vi "ComponentSimulatorA.vi"(8 "error in":errorcluster, 10 "ServerConfiguration":T1={"cmdServerPort"=8888, "telServerPort"=8889, "timeoutServerInMs"=100, "serverBytesToRead"=32768, "maxSizeQueueTcpClientFromDds"=1000, "EnqueueOptions"=enum."lossy enqueue", "timeoutQueueTcpClientFromDds (ms)"=50, "maxSizeQueueTcpClient"=1000, "timeoutInMs"=100}, 11 "tcpServer in":refnum<class "TcpServer.lvclass">) -> (0 "error out":errorcluster)   [LabVIEW 2018]
doc: "Simulate a software component that will use the TCP Server."
uses:
  src/TcpServerTel/typedef/queueOptionsTypeDef.ctl
  src/TcpServerTel/typedef/enqueueOptionsTypeDef.ctl
  src/TcpServer/configServerTypeDef.ctl
  src/TcpServer/TcpServer.lvclass
  src/TcpServerTel/typedef/telTypeDef.ctl
  src/TcpServer/TcpServer.lvclass/TcpServer.ctl
  src/TcpServerTel/TcpServerTel.lvclass/TcpServerTel.ctl
  src/TcpServer/runServer.vi
  src/TcpServerTel/TcpServerTel.lvclass
panel:
  out "Generic Message":string
  out "Clients Connected":bool
  in  "Telemetry Options":T3={"EnqueueOptions"=enum."lossy enqueue", "Timeout (ms)"=50}
  in  "Telemetry Timeout (ms)":i32=50
  out "Remaining Elements":i32
  out "One instance telemetry":string
  in  "getOneInstance":bool
  out "Telemetry Flushed":string[](array[string])
  in  "getQueueSize":bool
  out "Queue Size":i32
  in  "flushQueueFromDds":bool
  out "Event Received":string
  out "Command Received":string
  in  "Tab Control":T4(tab)
  out "ServerConfiguration":T1={"cmdServerPort"=8888, "telServerPort"=8889, "timeoutServerInMs"=100, "serverBytesToRead"=32768, "maxSizeQueueTcpClientFromDds"=1000, "EnqueueOptions"=enum."lossy enqueue", "timeoutQueueTcpClientFromDds (ms)"=50, "maxSizeQueueTcpClient"=1000, "timeoutInMs"=100}
  in  "fail":bool
  in  "success":bool
  in  "send_event":bool
  in  "Event Id":string="move"
  in  "Event Details":string="\"InPosition\" : true\n\n\"Tolerance\" : 0.2"
  in  "flushQueueToDds":bool
  in  "isQueueFull":bool
  in  "publish_telemetry":bool
  in  "send_telemetry":bool
  in  "Frecuency (cycles/s)":dbl=10.0
  in  "Duration (s)":dbl=2.0
  out "queueToDds":bool
  in  "Telemetry":T5={"Telemetry Id"="elevation", "telDetails"="\"compName\":\"MTMount\""}
  in  "stop_server":bool
  in  "Stop Simulator":bool caption="stop"
  # "Component Simulator A"
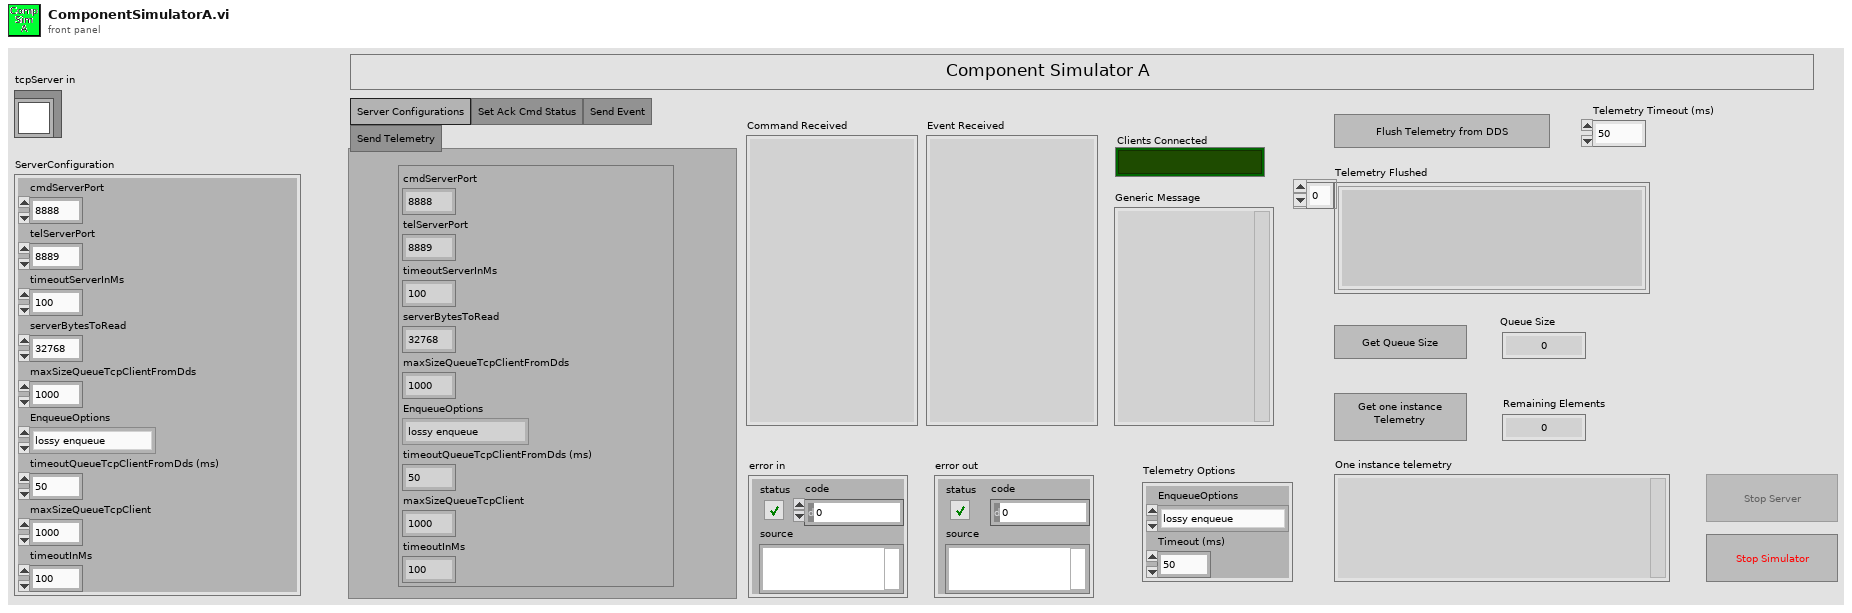
[diagram p1: front panel]
types:
  T1 = typedef "TcpServer.lvclass/configServerTypeDef.ctl" = cluster{"cmdServerPort":u16, "telServerPort":u16, "timeoutServerInMs":i32, "serverBytesToRead":i32, "maxSizeQueueTcpClientFromDds":i32, "EnqueueOptions":T2, "timeoutQueueTcpClientFromDds (ms)":i32, "maxSizeQueueTcpClient":i32, "timeoutInMs":i32}
  T2 = typedef "TcpServerTel.lvclass/enqueueOptionsTypeDef.ctl" = enum16{"lossy enqueue", "normal enqueue"}
  T3 = typedef "TcpServerTel.lvclass/queueOptionsTypeDef.ctl" = cluster{"EnqueueOptions":T2, "Timeout (ms)":i32}
  T4 = enum32{"Server Configurations", "Set Ack Cmd Status", "Send Event", "Send Telemetry"}
  T5 = cluster{"Telemetry Id":string, "telDetails":string}
  T6 = typedef "TcpServerTel.lvclass/telTypeDef.ctl" = cluster{"name":string, "telDetails":string}
  T7 = enum16{"queueTcpClientFromDds", "queueTcpClient"}
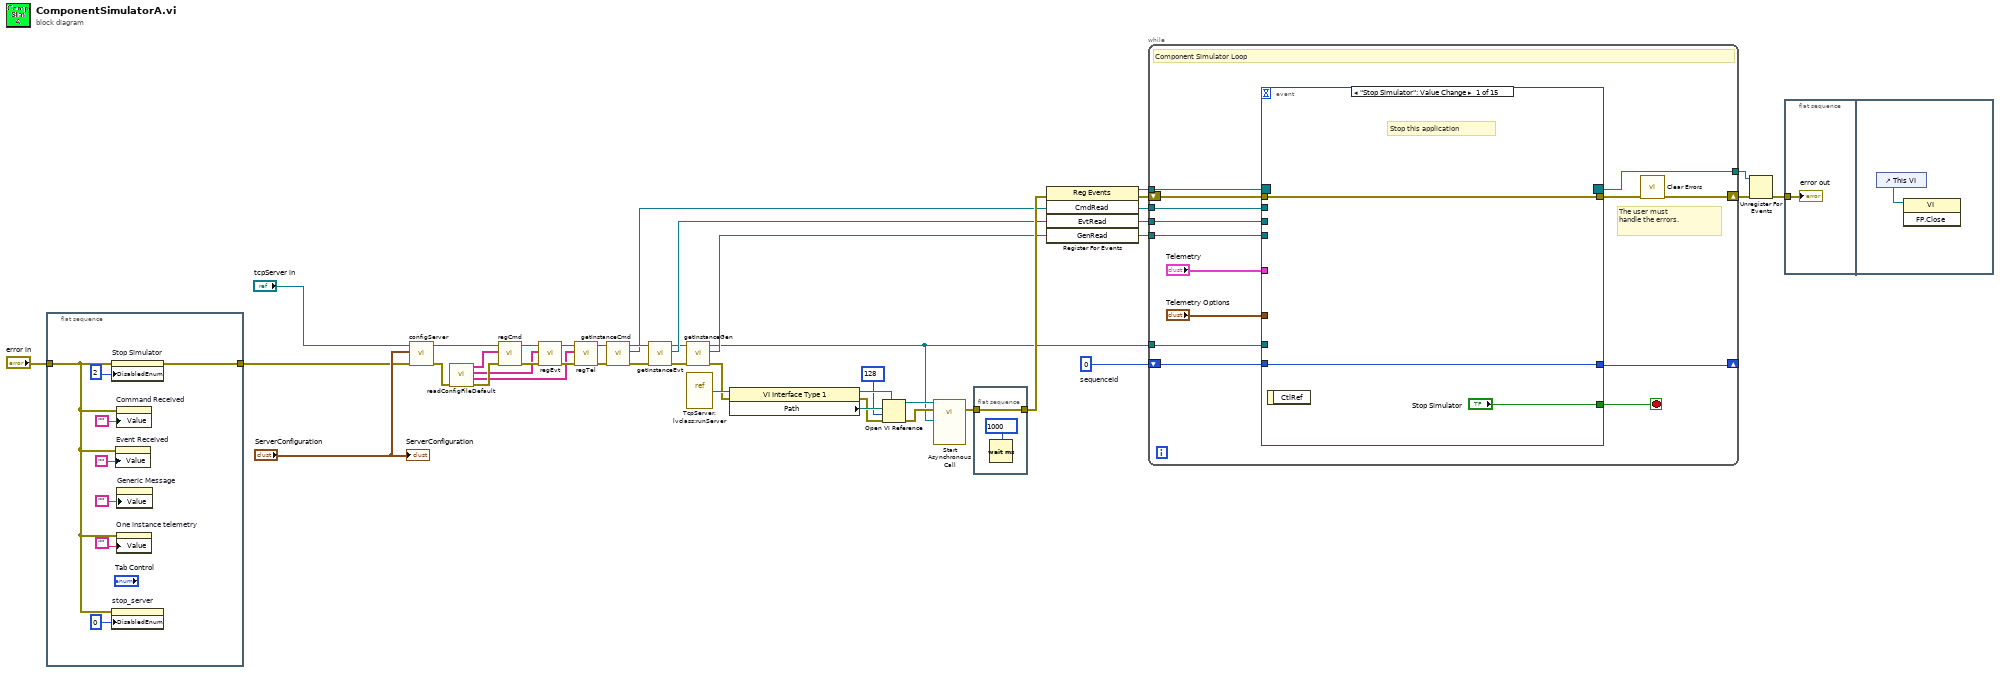
[diagram p0: block diagram]
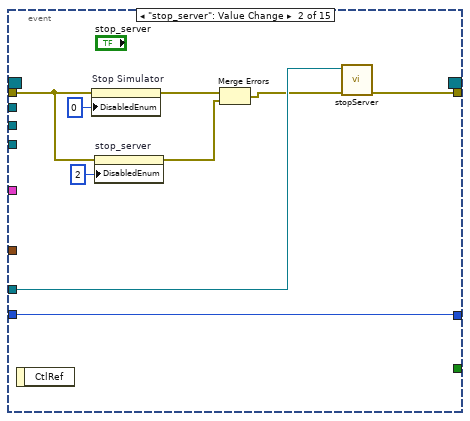
[diagram p2: hidden frame]
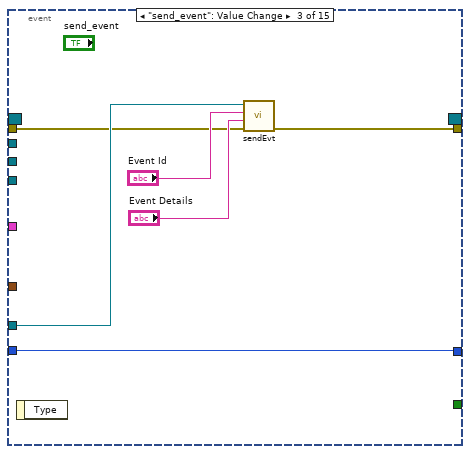
[diagram p3: hidden frame]
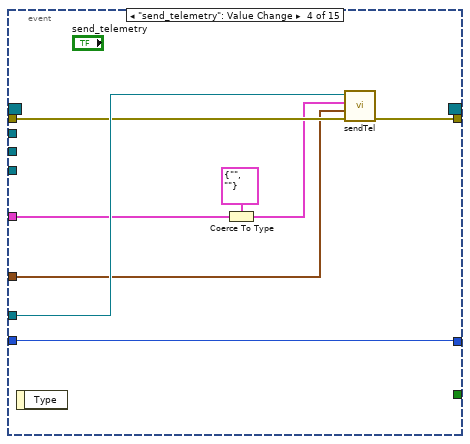
[diagram p4: hidden frame]
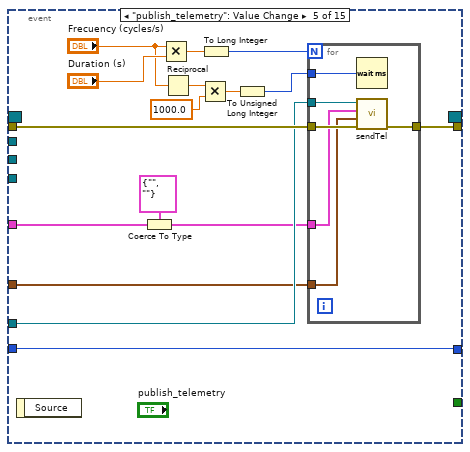
[diagram p5: hidden frame]
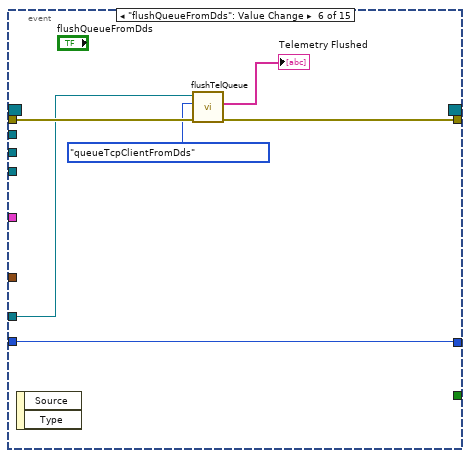
[diagram p6: hidden frame]
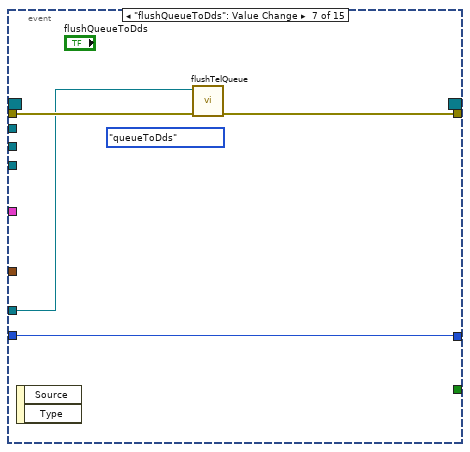
[diagram p7: hidden frame]
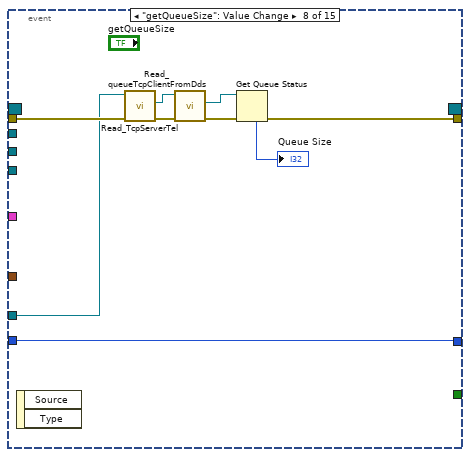
[diagram p8: hidden frame]
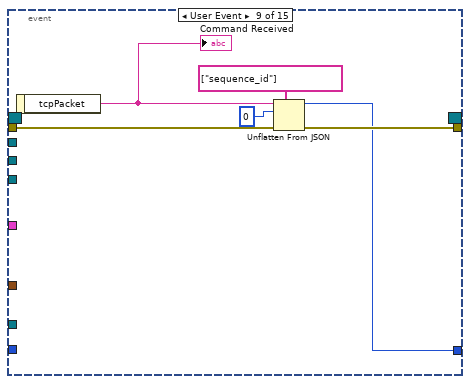
[diagram p9: hidden frame]
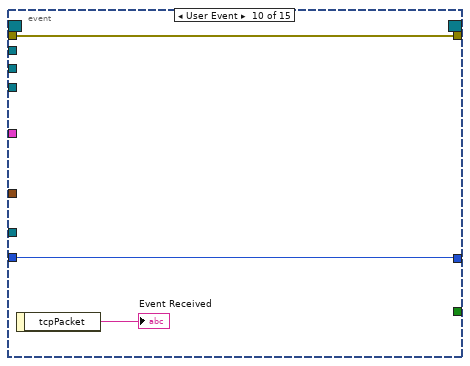
[diagram p10: hidden frame]
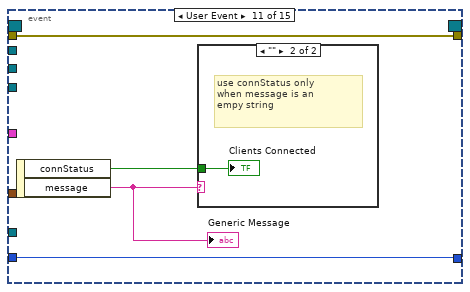
[diagram p11: hidden frame]
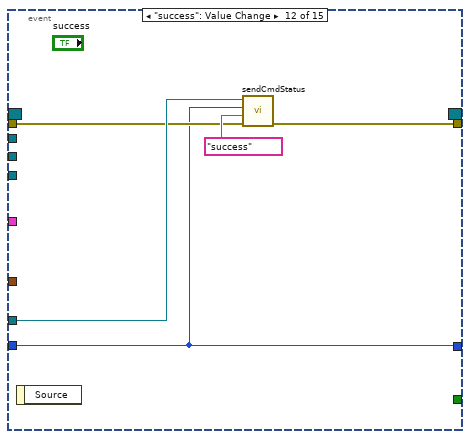
[diagram p13: hidden frame]
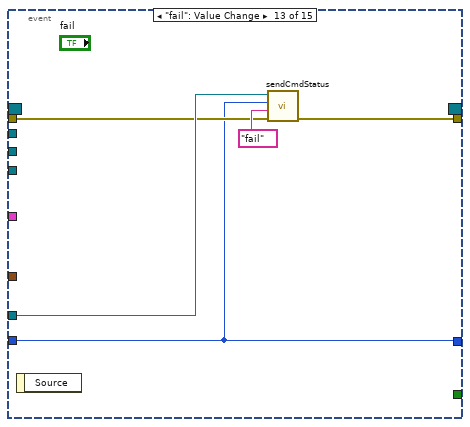
[diagram p14: hidden frame]
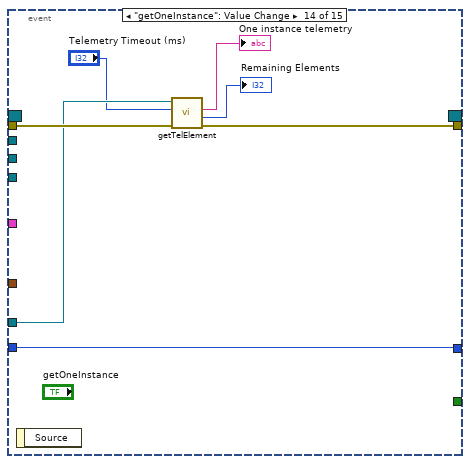
[diagram p15: hidden frame]
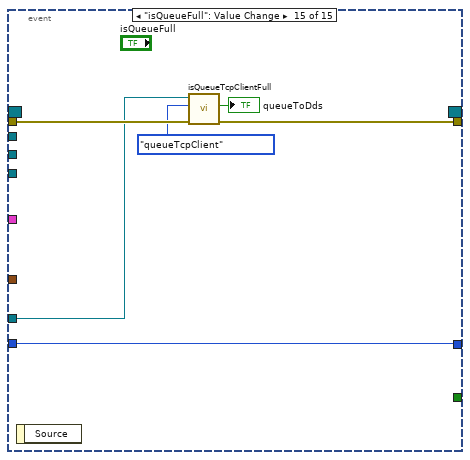
[diagram p16: hidden frame]
diagram:
  w5 = 0  # sequenceId
  n1 = flat-sequence {
    tunnel: "error in" -> [w43]
    tunnel: [w47] -> w2
    frame #0 {
      n2 = property on="Stop Simulator" class="Bool"(error in=w43, "DisabledEnum"=2) -> (error out=w47:errorcluster)  [unwired: 1 in, 1 out]
      n3 = property on="stop_server" class="Bool"(error in=w43, "DisabledEnum"=0) -> ()  [unwired: 1 in, 2 out]
      n4 = property on="Event Received" class="Str"(error in=w43, "Value"="") -> ()  [unwired: 1 in, 2 out]
      n5 = property on="Command Received" class="Str"(error in=w43, "Value"="") -> ()  [unwired: 1 in, 2 out]
      n6 = property on="One instance telemetry" class="Str"(error in=w43, "Value"="") -> ()  [unwired: 1 in, 2 out]
      n7 = property on="Generic Message" class="Str"("Value"="") -> ()  [unwired: 2 in, 2 out]
    }
  }
  n8 = call "configServer.vi"("error in (no error)"=w2, "ServerConfiguration"="ServerConfiguration", "tcpServer in"="tcpServer in") -> ("error out"=w14:errorcluster, "tcpServer out"=w37:refnum<class "TcpServer.lvclass">)  [unwired: 7 in]
  n9 = call "readConfigFileDefault.vi"("error in (no error)"=w14) -> ("error out"=w13:errorcluster, "regTel"=w7:string[][], "regEvt"=w11:string[][], "regCmd"=w12:string[])  [unwired: 7 in]
  n10 = call "regCmd.vi"("error in (no error)"=w13, "cmdReg"=w12, "tcpServer in"=w37) -> ("error out"=w38:errorcluster, "tcpServer out"=w18:refnum<class "TcpServer.lvclass">)  [unwired: 7 in]
  n11 = call "regEvt.vi"("error in (no error)"=w38, "evtReg"=w11, "tcpServer in"=w18) -> ("error out"=w19:errorcluster, "tcpServer out"=w9:refnum<class "TcpServer.lvclass">)  [unwired: 7 in]
  n12 = call "regTel.vi"("error in (no error)"=w19, "telReg"=w7, "tcpServer in"=w9) -> ("error out"=w10:errorcluster, "tcpServer out"=w8:refnum<class "TcpServer.lvclass">)  [unwired: 7 in]
  n13 = call "getInstanceCmd.vi"("error in (no error)"=w10, "tcpServer in"=w8) -> ("error out"=w36:errorcluster, "CmdRead"=w22:refnum<user-event>, "tcpServer out"=w34:refnum<class "TcpServer.lvclass">)  [unwired: 7 in]
  n14 = call "getInstanceEvt.vi"("error in (no error)"=w36, "tcpServer in"=w34) -> ("error out"=w35:errorcluster, "EvtRead"=w21:refnum<user-event>, "tcpServer out"=w16:refnum<class "TcpServer.lvclass">)  [unwired: 7 in]
  n15 = call "getInstanceGen.vi"("error in (no error)"=w35, "tcpServer in"=w16) -> ("error out"=w17:errorcluster, "GenRead"=w15:refnum<user-event>, "tcpServer out"=w6:refnum<class "TcpServer.lvclass">)  [unwired: 7 in]
  n16 = vi-ref "TcpServer.lvclass:runServer.vi"() -> (w33:refnum<vi>)
  n17 = property class="VI Interface Type 1"(reference=w33, error in=w17) -> (reference out=w31:refnum<vi>, error out=w28:errorcluster, "Path"=w32:path)
  n18 = Open VI Reference(type specifier VI Refnum (for type only)=w31, vi path=w32, options=128, error in (no error)=w28) -> (vi reference=w29:refnum<vi>, error out=w27:errorcluster)  [unwired: 2 in]
  n19 = call-by-ref "Start Asynchronous Call"(reference=w29, error in=w27, "TcpServer in"=w6) -> (error out=w26:errorcluster)  [unwired: 9 in, 3 out]
  n20 = flat-sequence {
    tunnel: w26 -> [w49]
    tunnel: [w49] -> w25
    frame #0 {
      n21 = Wait (ms)(milliseconds to wait=u32 1000) -> ()  [unwired: 1 out]
    }
  }
  n22 = register-events(error in=w25, w22, w21, w15) -> (reference out=w40:refnum<event-registration>, error out=w39:errorcluster)  [unwired: 1 in]
  n23 = while {
    tunnel: w40 -> [w63]
    shift-right: [w62] -> _
    shift-left: w5 -> [w61]
    shift-right: [w51] -> w24
    shift-left: w39 -> [w64]
    tunnel: [w59] -> w23
    tunnel: w22 -> [w58]
    tunnel: w21 -> [w57]
    tunnel: w15 -> [w56]
    tunnel: w6 -> [w55]
    stop <- w52 stop-if-true
    # "The user must\nhandle the errors."
    # "Component Simulator Loop"
    n24 = event shown="[0] \"Stop Simulator\": Value Change" {
      selector: w63 -> [_ _ _ _ _ _ _ _ _ _ _ _ _ _ _]
      dyn-events: [_ _ _ _ _ _ _ _ _ _ _ _ _ _ _] -> w59
      timeout: _ -> [_ _ _ _ _ _ _ _ _ _ _ _ _ _ _]
      tunnel: ["Stop Simulator" _ _ _ _ _ _ _ _ _ _ _ _ _ _] -> w52
      tunnel: [w66 w68 w78 w88 w101 w115 w119 w123 w134 w140 w144 w149 w154 w157 w164] -> w60
      tunnel: w64 -> [w66 w72 w77 w87 w102 w117 w121 w128 w135 w140 w144 w147 w152 w161 w166]
      tunnel: [w65 w76 w82 w90 w106 w118 w122 w131 w132 w139 w143 w146 w151 w162 w168] -> w62
      tunnel: w61 -> [w65 w76 w82 w90 w106 w118 w122 w131 _ w139 w143 w146 w151 w162 w168]
      tunnel: w58 -> [_ _ _ _ _ _ _ _ _ _ _ _ _ _ _]
      tunnel: w57 -> [_ _ _ _ _ _ _ _ _ _ _ _ _ _ _]
      tunnel: w56 -> [_ _ _ _ _ _ _ _ _ _ _ _ _ _ _]
      tunnel: w55 -> [_ w75 w81 w89 w95 w116 w120 w127 _ _ _ w148 w153 w160 w165]
      tunnel: "Telemetry" -> [_ _ _ w86 w93 _ _ _ _ _ _ _ _ _ _]
      tunnel: "Telemetry Options" -> [_ _ _ w83 w91 _ _ _ _ _ _ _ _ _ _]
      event "Stop Simulator": Value Change {
        # "Stop this application"
        n25 = event-data() -> ()  [unwired: 1 in, 1 out]
      }
      event "stop_server": Value Change {
        n26 = event-data() -> ()  [unwired: 1 in, 1 out]
        n27 = property on="Stop Simulator" class="Bool"(error in=w72, "DisabledEnum"=0) -> (error out=w71:errorcluster)  [unwired: 1 in, 1 out]
        n28 = property on="stop_server" class="Bool"(error in=w72, "DisabledEnum"=2) -> (error out=w70:errorcluster)  [unwired: 1 in, 1 out]
        n29 = Merge Errors(w71, w70) -> (w69:errorcluster)
        n30 = call "stopServer.vi"("error in (no error)"=w69, "tcpServer in"=w75) -> ("error out"=w68:errorcluster)  [unwired: 8 in, 1 out]
      }
      event "send_event": Value Change {
        n31 = event-data() -> ()  [unwired: 1 in, 1 out]
        n32 = call "sendEvt.vi"("error in (no error)"=w77, "Event Details"="Event Details", "Event Id"="Event Id", "tcpServer in"=w81) -> ("error out"=w78:errorcluster)  [unwired: 6 in, 1 out]
      }
      event "send_telemetry": Value Change {
        n33 = event-data() -> ()  [unwired: 1 in, 1 out]
        n34 = Coerce To Type(0:w86, 1:T6 {"name"="", "telDetails"=""} ("Telemetry")) -> (2:w85:T6)
        n35 = call "sendTel.vi"("error in (no error)"=w87, "queueOptions"=w83, "Telemetry"=w85, "tcpServer in"=w89) -> ("error out"=w88:errorcluster)  [unwired: 6 in, 1 out]
      }
      event "publish_telemetry": Value Change {
        n36 = event-data() -> ()  [unwired: 1 in, 1 out]
        n37 = Coerce To Type(0:w93, 1:T6 {"name"="", "telDetails"=""} ("Telemetry")) -> (2:w92:T6)
        n38 = Multiply(x="Frecuency (cycles/s)", y="Duration (s)") -> (x*y=w104:dbl)
        n39 = Reciprocal(x="Frecuency (cycles/s)") -> (1/x=w99:dbl)
        n40 = Multiply(x=w99, y=1000.0) -> (x*y=w97:dbl)
        n41 = To Long Integer(number=w104) -> (32bit integer=w103:i32)
        n42 = To Unsigned Long Integer(number=w97) -> (unsigned 32bit integer=w96:u32)
        n43 = for {
          N: w103 -> [_]
          tunnel: w102 -> [w112]
          tunnel: [w107] -> w101
          tunnel: w96 -> [w111]
          tunnel: w95 -> [w110]
          tunnel: w92 -> [w109]
          tunnel: w91 -> [w108]
          n44 = Wait (ms)(milliseconds to wait=w111) -> ()  [unwired: 1 out]
          n45 = call "sendTel.vi"("error in (no error)"=w112, "queueOptions"=w108, "Telemetry"=w109, "tcpServer in"=w110) -> ("error out"=w107:errorcluster)  [unwired: 6 in, 1 out]
        }
      }
      event "flushQueueFromDds": Value Change {
        n46 = event-data() -> ()  [unwired: 1 in, 2 out]
        n47 = call "flushTelQueue.vi"("error in (no error)"=w117, "queueName"=T7."queueTcpClientFromDds", "TcpServer in"=w116) -> ("error out"=w115:errorcluster, "telemetry flushed"=→"Telemetry Flushed":string[])  [unwired: 6 in, 1 out]
      }
      event "flushQueueToDds": Value Change {
        (unwired) enum16{"queueFromDds", "queueToDds"}."queueToDds" ("queueName")
        n48 = event-data() -> ()  [unwired: 1 in, 2 out]
        n49 = call "flushTelQueue.vi"("error in (no error)"=w121, "TcpServer in"=w120) -> ("error out"=w119:errorcluster)  [unwired: 7 in, 2 out]
      }
      event "getQueueSize": Value Change {
        n50 = event-data() -> ()  [unwired: 1 in, 2 out]
        n51 = call "Read_TcpServerTel.vi"("error in (no error)"=w128, "TcpServer in"=w127) -> ("error out"=w129:errorcluster, "TcpServerTel.lvclass"=w130:refnum<class "TcpServerTel.lvclass">)  [unwired: 7 in, 1 out]
        n52 = call "Read_queueTcpClientFromDds.vi"("error in (no error)"=w129, "TcpServerTel in"=w130) -> ("error out"=w126:errorcluster, "queueTcpClientFromDds"=w125:refnum<queue>)  [unwired: 7 in, 1 out]
        n53 = Get Queue Status(queue=w125, error in (no error)=w126) -> (error out=w123:errorcluster, # elements in queue=→"Queue Size":i32)  [unwired: 1 in, 6 out]
      }
      event User Event {
        n54 = event-data() -> ("tcpPacket"=w133:string)  [unwired: 1 in]
        "Command Received" <- w133
        n55 = Unflatten From JSON(path=string[] ["sequence_id"], JSON string=w133, type and defaults=0, error in (no error)=w135) -> (value=w132:i32, error out=w134:errorcluster)  [unwired: 3 in]
      }
      event User Event {
        n56 = event-data() -> ("tcpPacket"=→"Event Received":string)  [unwired: 1 in]
      }
      event User Event {
        n57 = event-data() -> ("connStatus"=w142:bool, "message"=w141:string)  [unwired: 1 in]
        "Generic Message" <- w141
        n58 = case shown="\"\"" w141 {
          tunnel: w142 -> [_ w145]
          frame Default {
          }
          frame "" {
            # "use connStatus only\nwhen message is an\nempy string"
            "Clients Connected" <- w145
          }
        }
      }
      event "success": Value Change {
        n59 = event-data() -> ()  [unwired: 1 in, 1 out]
        n60 = call "sendCmdStatus.vi"("error in (no error)"=w147, "cmdStatus"="success", "sequenceId"=w146, "tcpServer in"=w148) -> ("error out"=w149:errorcluster)  [unwired: 6 in, 1 out]
      }
      event "fail": Value Change {
        n61 = event-data() -> ()  [unwired: 1 in, 1 out]
        n62 = call "sendCmdStatus.vi"("error in (no error)"=w152, "cmdStatus"="fail", "sequenceId"=w151, "tcpServer in"=w153) -> ("error out"=w154:errorcluster)  [unwired: 6 in, 1 out]
      }
      event "getOneInstance": Value Change {
        n63 = event-data() -> ()  [unwired: 1 in, 1 out]
        n64 = call "getTelElement.vi"("error in (no error)"=w161, "timeoutQueueTcpClientFromDds"="Telemetry Timeout (ms)", "TcpServer in"=w160) -> ("error out"=w157:errorcluster, "Remaining Elements"=→"Remaining Elements":i32, "tcpPacket"=→"One instance telemetry":string)  [unwired: 5 in, 1 out]
      }
      event "isQueueFull": Value Change {
        n65 = event-data() -> ()  [unwired: 1 in, 1 out]
        n66 = call "isQueueTcpClientFull.vi"("error in (no error)"=w166, "queueName"=T7."queueTcpClient", "tcpServer in"=w165) -> ("error out"=w164:errorcluster, "queueFull"=→"queueToDds":bool)  [unwired: 6 in, 1 out]
      }
    }
    n67 = call <vilib>:"Clear Errors.vi"("error in (no error)"=w60) -> ("error out"=w51:errorcluster)  [unwired: 5 in, 1 out]
  }
  n68 = Unregister For Events(event registration refnum=w23, error in=w24) -> (error out=w3:errorcluster)
  n69 = flat-sequence {
    tunnel: w3 -> [w169]
    frame #0 {
      "error out" <- w169
    }
    frame #1 {
      n70 = control-ref of="This VI"() -> (w170:refnum<vi>)
      n71 = invoke class="VI" method="FP.Close"(reference=w170) -> ()  [unwired: 2 in, 3 out]
    }
  }
  "ServerConfiguration" <- "ServerConfiguration"
